vi "FlushQueueMessage.vi"(8 "error in":errorcluster, 11 "message ref in":refnum<class "CLM_LocalMessage_Queue.lvclass">) -> (0 "error out":errorcluster, 2 "remaining elements":T1[](array[typedef]), 3 "message ref out out":refnum<class "CLM_LocalMessage_Queue.lvclass">)   [LabVIEW 2013, in "CLM_LocalMessage_Queue.lvclass"]
uses:
  CLM_LocalMessage_Queue.lvclass
  LocalMessage/Message.ctl
  CLM_LocalMessage_Queue.lvclass/CLM_LocalMessage_Queue.ctl
  LocalMessage/CLM_LocalMessage.lvclass
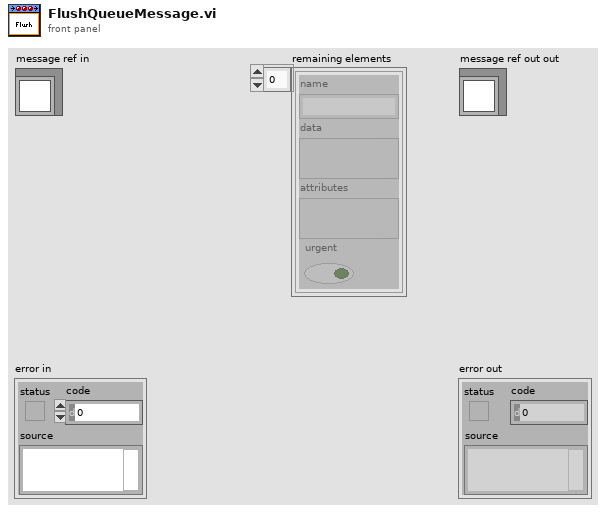
[diagram p1: front panel]
types:
  T1 = typedef "CLM_LocalMessage.lvclass/Message.ctl" = cluster{"name":string, "data":variant, "attributes":variant, "urgent":bool}
  T2 = typedef "CLM_LocalMessage_Queue.lvclass/MessageQueue.ctl" = refnum<queue>
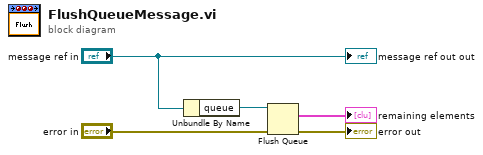
[diagram p0: block diagram]
diagram:
  n1 = Unbundle By Name("message ref in") -> ("queue"=w4:T2)
  n2 = Flush Queue(queue=w4, error in (no error)="error in") -> (remaining elements=→"remaining elements":T1[], error out=→"error out":errorcluster)  [unwired: 1 out]
  "message ref out out" <- "message ref in"
